vi "Set Mask.vi"(8 "error in (no error)":errorcluster, 9 "Alpha (255)":i32=255, 10 "Mask Color (Cyan)":u32(colorbox)=65535, 11 "VI Ref In":refnum<vi>) -> (0 "error out":errorcluster, 3 "VI Ref Out":refnum<vi>)   [LabVIEW 2019, in "Window.lvlib"]
doc: "Set a color mask and opacity for the given VI's front panel. Will make the mask color transparent, while setting the overall window's transparency.\n\nNOTE: LabVIEW's Transprency setting for a front panel will reset the window mask."
uses:
  Window.lvlib
  User32.dll
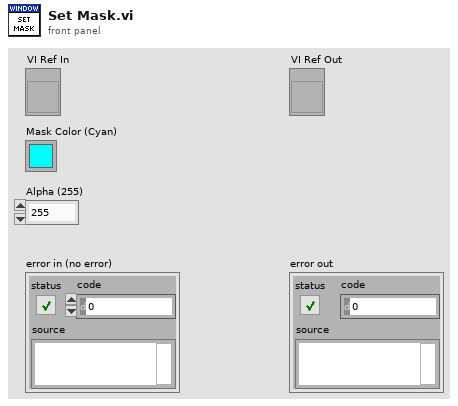
[diagram p1: front panel]
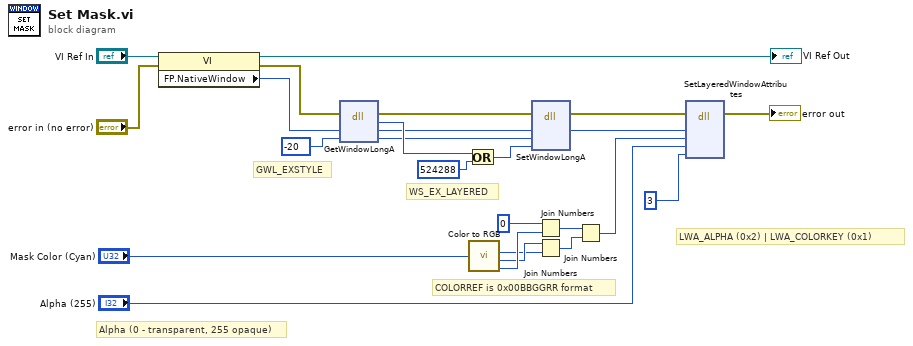
[diagram p0: block diagram]
diagram:
  # "LWA_ALPHA (0x2) | LWA_COLORKEY (0x1)"
  # "COLORREF is 0x00BBGGRR format"
  # "WS_EX_LAYERED"
  # "GWL_EXSTYLE"
  # "Alpha (0 - transparent, 255 opaque)"
  n1 = property class="VI"(reference="VI Ref In", error in="error in (no error)") -> (reference out=→"VI Ref Out":refnum<vi>, error out=w1:errorcluster, "FP.NativeWindow"=w2:u64)
  n2 = dll-call lib="USER32.DLL" fn="GetWindowLongA"(error in=w1, "handle"=w2, "nIndex"=-20) -> (error out=w19:errorcluster, w23:i32, "handle"=w16:i32, "nIndex"=w18:i32)  [unwired: 2 in, 1 out]
  n3 = Or(x=w23, y=524288) -> (x .or. y?=w25:i32)
  n4 = call <vilib>:"Color to RGB.vi"("Color"="Mask Color (Cyan)") -> ("R"=w11:u8, "G"=w12:u8, "B"=w13:u8)  [unwired: 1 out]
  n5 = dll-call lib="USER32.DLL" fn="SetWindowLongA"(error in=w19, "handle"=w16, "nIndex"=w18, "dwNewLong"=w25) -> (error out=w17:errorcluster, "handle"=w15:i32)  [unwired: 4 in, 2 out]
  n6 = Join Numbers(hi=u8 0, lo=w13) -> ((hi.lo)=w10:u16)
  n7 = Join Numbers(hi=w12, lo=w11) -> ((hi.lo)=w9:u16)
  n8 = Join Numbers(hi=w10, lo=w9) -> ((hi.lo)=w8:u32)
  n9 = dll-call lib="USER32.DLL" fn="SetLayeredWindowAttributes"(error in=w17, "handle"=w15, "crkey"=w8, "bAlpha"="Alpha (255)", "dwFlags"=3) -> (error out=→"error out":errorcluster)  [unwired: 6 in, 2 out]
